vi "速度轉電壓 三軸平台 Axis 3.vi"(1 "Speed (0.1mm/s)":fxp<+/-,64,32>) -> (0 "Voltage\nOutput":fxp<+/-,64,32>)   [LabVIEW 2019]
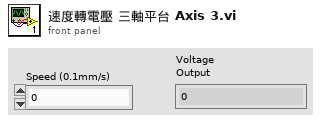
[diagram p1: front panel]
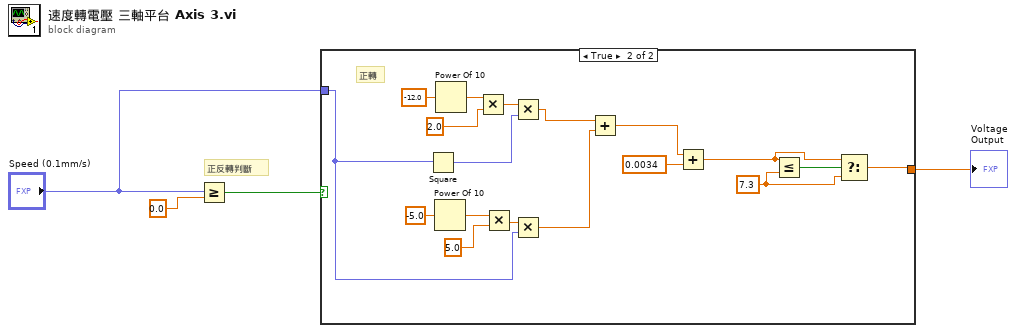
[diagram p0: block diagram]
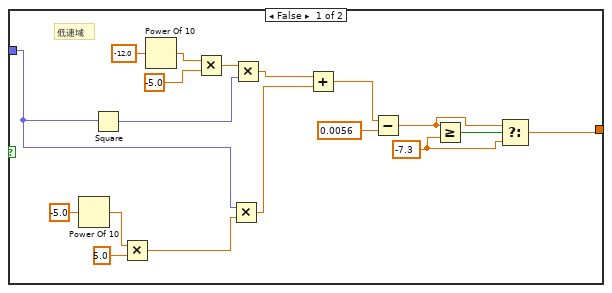
[diagram p2: hidden frame]
diagram:
  # "正反轉判斷"
  n1 = Greater Or Equal?(x="Speed (0.1mm/s)", y=0.0) -> (x >= y?=w3:bool)
  n2 = case shown="True" w3 {
    tunnel: "Speed (0.1mm/s)" -> [w10 w31]
    tunnel: [w6 w24] -> w1
    frame False {
      w5 = -7.3 ("y")
      # "低速域"
      n3 = Power Of 10(x=-5.0) -> (10^x=w13:dbl)
      n4 = Square(x=w10) -> (x^2=w18:fxp<+,64,63>)
      n5 = Multiply(x=w13, y=5.0) -> (x*y=w11:dbl)
      n6 = Power Of 10(x=-12.0) -> (10^x=w21:dbl)
      n7 = Multiply(x=w21, y=-5.0) -> (x*y=w19:dbl)
      n8 = Multiply(x=w10, y=w11) -> (x*y=w9:dbl)
      n9 = Multiply(x=w19, y=w18) -> (x*y=w17:dbl)
      n10 = Add(x=w17, y=w9) -> (x+y=w16:dbl)
      n11 = Subtract(x=w16, y=0.0056) -> (x-y=w7:dbl)
      n12 = Greater Or Equal?(x=w7, y=w5) -> (x >= y?=w8:bool)
      n13 = Select(t=w7, s=w8, f=w5) -> (s? t:f=w6:dbl)
    }
    frame True {
      w23 = 7.3 ("y")
      # "正轉"
      n14 = Square(x=w31) -> (x^2=w36:fxp<+,64,63>)
      n15 = Power Of 10(x=-5.0) -> (10^x=w34:dbl)
      n16 = Power Of 10(x=-12.0) -> (10^x=w39:dbl)
      n17 = Multiply(x=w39, y=2.0) -> (x*y=w37:dbl)
      n18 = Multiply(x=w34, y=5.0) -> (x*y=w32:dbl)
      n19 = Multiply(x=w37, y=w36) -> (x*y=w30:dbl)
      n20 = Multiply(x=w32, y=w31) -> (x*y=w29:dbl)
      n21 = Add(x=w30, y=w29) -> (x+y=w28:dbl)
      n22 = Add(x=w28, y=0.0034) -> (x+y=w25:dbl)
      n23 = Less Or Equal?(x=w25, y=w23) -> (x <= y?=w26:bool)
      n24 = Select(t=w25, s=w26, f=w23) -> (s? t:f=w24:dbl)
    }
  }
  "Voltage\nOutput" <- w1
